vi "Agilent N6700 Series Configure Voltage.vi"() -> ()   [LabVIEW 2021]
doc: "Configures the power supply's output range on a channel, configures the DC voltage level, channel appears at the output connector and takes a measurement on the output signal and returns the measured value."
uses:
  <instrlib>/Agilent N6700 Series/Agilent N6700 Series.lvlib
panel:
  in  "error in":errorcluster {"code" format="%.0x"}
  out "error out":errorcluster {"code" format="%.0x"}
  in  "Current Limit":dbl=1.0 format="%^.3e"
  in  "Behavior":i32(ring) items=["Regulatory Limit", "Trip Limit"]
  out "Voltage Measurement":dbl format="%^.3e"
  in  "Voltage Level":dbl=5.0 format="%^.3e"
  in  "Voltage Range":dbl=10.0 format="%^.3e"
  in  "Agilent SMUChannel":string="1"
  in  "Agilent SMU":refnum<visa-resource-name>
  # "Agilent N6700 DC Power Supply"
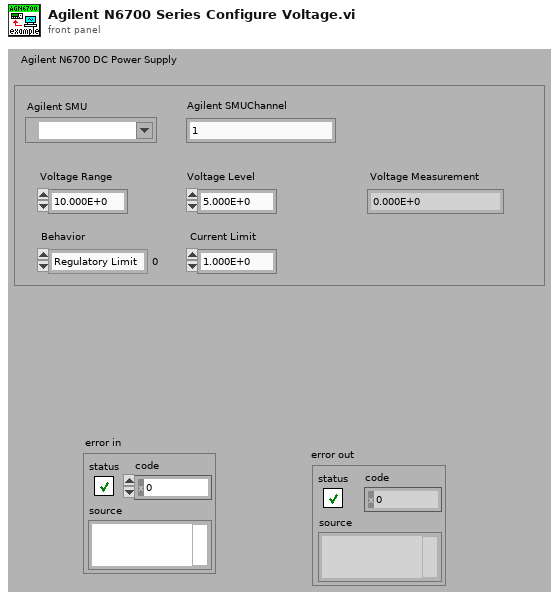
[diagram p1: front panel]
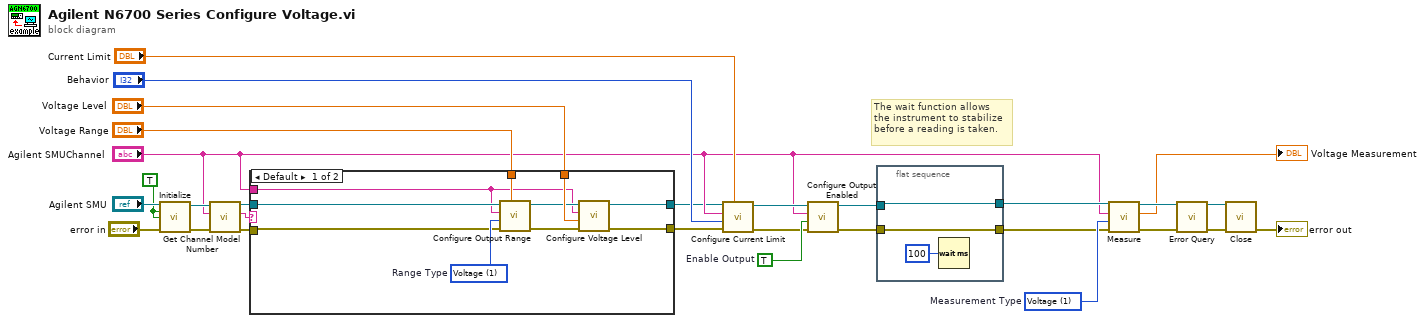
[diagram p0: block diagram]
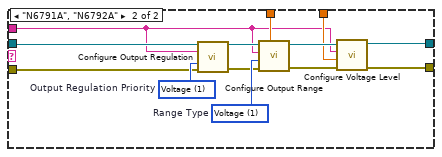
[diagram p2: hidden frame]
diagram:
  w20 = TRUE ("Reset? (T: Yes)")
  w21 = 1 items=["Voltage"=1, "Current"=0]  # Measurement Type
  w22 = TRUE  # Enable Output
  # "The wait function allows \nthe instrument to stabilize\nbefore a reading is taken."
  n1 = call <instrlib>:"Initialize.vi"("VISA resource name"="Agilent SMU", "ID Query? (T: Yes)"=w20, "Reset? (T: Yes)"=w20, "error in (no error)"="error in") -> ("VISA resource name out"=w11:refnum<visa-resource-name>, "error out"=w10:errorcluster)  [unwired: 10 in]
  n2 = call <instrlib>:"Get Channel Model Number.vi"("error in (no error)"=w10, "Channel Name (1)"="Agilent SMUChannel", "VISA resource name"=w11) -> ("error out"=w8:errorcluster, "Model Number"=w7:string, "VISA resource name out"=w9:refnum<visa-resource-name>)  [unwired: 6 in]
  n3 = case shown="Default" w7 {
    tunnel: "Voltage Range" -> [w36 w52]
    tunnel: "Agilent SMUChannel" -> [w30 w42]
    tunnel: w9 -> [w38 w47]
    tunnel: w8 -> [w37 w46]
    tunnel: "Voltage Level" -> [w34 w43]
    tunnel: [w32 w40] -> w4
    tunnel: [w31 w41] -> w3
    frame Default {
      w39 = 1 items=["Voltage"=1, "Current"=0]  # Range Type
      n4 = call <instrlib>:"Configure Output Range.vi"("Range (0.0)"=w36, "error in (no error)"=w37, "Range Type (1: Voltage)"=w39, "Channel Name (1)"=w30, "VISA resource name"=w38) -> ("error out"=w35:errorcluster, "VISA resource name out"=w33:refnum<visa-resource-name>)  [unwired: 5 in]
      n5 = call <instrlib>:"Configure Voltage Level.vi"("error in (no error)"=w35, "Level  (0.0 volts)"=w34, "Channel Name (1)"=w30, "VISA resource name"=w33) -> ("error out"=w32:errorcluster, "VISA resource name out"=w31:refnum<visa-resource-name>)  [unwired: 6 in]
    }
    frame "N6791A", "N6792A" {
      w48 = 1 items=["Voltage"=1, "Current"=0]  # Output Regulation Priority
      w51 = 1 items=["Voltage"=1, "Current"=0]  # Range Type
      n6 = call <instrlib>:"Configure Output Regulation.vi"("VISA resource name"=w47, "Channel Name (1)"=w42, "Output Regulation Priority (1: Voltage)"=w48, "error in (no error)"=w46) -> ("VISA resource name out"=w50:refnum<visa-resource-name>, "error out"=w49:errorcluster)  [unwired: 10 in]
      n7 = call <instrlib>:"Configure Output Range.vi"("Range (0.0)"=w52, "error in (no error)"=w49, "Range Type (1: Voltage)"=w51, "Channel Name (1)"=w42, "VISA resource name"=w50) -> ("error out"=w44:errorcluster, "VISA resource name out"=w45:refnum<visa-resource-name>)  [unwired: 5 in]
      n8 = call <instrlib>:"Configure Voltage Level.vi"("error in (no error)"=w44, "Level  (0.0 volts)"=w43, "Channel Name (1)"=w42, "VISA resource name"=w45) -> ("error out"=w40:errorcluster, "VISA resource name out"=w41:refnum<visa-resource-name>)  [unwired: 6 in]
    }
  }
  n9 = call <instrlib>:"Configure Current Limit.vi"("Limit (0.0 amps)"="Current Limit", "error in (no error)"=w4, "Behavior (0: Regulatory Limit)"="Behavior", "Channel Name (1)"="Agilent SMUChannel", "VISA resource name"=w3) -> ("error out"=w19:errorcluster, "VISA resource name out"=w18:refnum<visa-resource-name>)  [unwired: 5 in]
  n10 = call <instrlib>:"Configure Output Enabled.vi"("error in (no error)"=w19, "Enable Output (False)"=w22, "Channel Name (1)"="Agilent SMUChannel", "VISA resource name"=w18) -> ("error out"=w12:errorcluster, "VISA resource name out"=w15:refnum<visa-resource-name>)  [unwired: 6 in]
  n11 = flat-sequence {
    tunnel: w15 -> [w55]
    tunnel: [w55] -> w14
    tunnel: [w53] -> w13
    tunnel: w12 -> [w53]
    frame #0 {
      n12 = Wait (ms)(milliseconds to wait=u32 100) -> ()  [unwired: 1 out]
    }
  }
  n13 = call <instrlib>:"Measure.vi"("error in (no error)"=w13, "Measurement Type (1: Voltage)"=w21, "Channel Name (1)"="Agilent SMUChannel", "VISA resource name"=w14) -> ("error out"=w29:errorcluster, "Measurement"=→"Voltage Measurement":dbl, "VISA resource name out"=w26:refnum<visa-resource-name>)  [unwired: 5 in]
  n14 = call <instrlib>:"Error Query.vi"("VISA resource name"=w26, "error in (no error)"=w29) -> ("VISA resource name out"=w27:refnum<visa-resource-name>, "error out"=w28:errorcluster)  [unwired: 10 in, 2 out]
  n15 = call <instrlib>:"Close.vi"("VISA resource name"=w27, "error in (no error)"=w28) -> ("error out"=→"error out":errorcluster)  [unwired: 13 in]
